vi "Check Amplitude Bin.vi"(1 "Threshold Amp":dbl, 3 "Max Amp":dbl) -> (0 "Check Amp Ok?":bool)   [LabVIEW 2014]
doc: "This subVI is used to check if the max amplitude of frequency bins is over the maximum noise amplitude threshold"
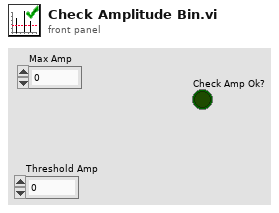
[diagram p1: front panel]
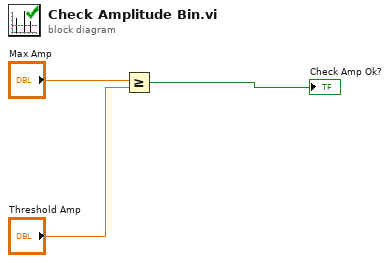
[diagram p0: block diagram]
diagram:
  n1 = Greater Or Equal?(x="Max Amp", y="Threshold Amp") -> (x >= y?=→"Check Amp Ok?":bool)
